vi "Timing Test.vi"() -> ()   [LabVIEW 2021]
uses:
  Ethernet/Ethernet.lvclass
  C:/Projects/1200-00006 _ BS1200/Engineering/Software/LabVIEW Driver/LV2021 Driver V2.0.0/BS1200 Driver/Battery Simulator 1200 Driver.lvclass
  CAN/CAN.lvclass
  Battery Simulator 1200 Driver.lvclass
panel:
  in  "Mode":enum16{"TCPIP", "CAN"}(ring)=enum."CAN"
  in  "CAN Interface":refnum<k21>="CAN1"
  out "Last update":timestamp
  in  "Stop Button":bool
  in  "UDP port":u16=54321
  in  "TCP port":u16=12345
  in  "Box IP address":string="192.168.1.100"
  in  "Update channel 1 voltage":dbl
  out "Array - String":string[](array[string])
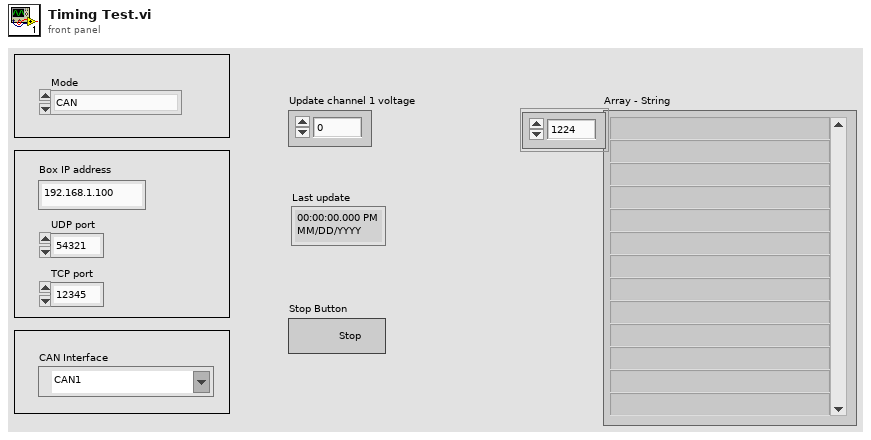
[diagram p1: front panel]
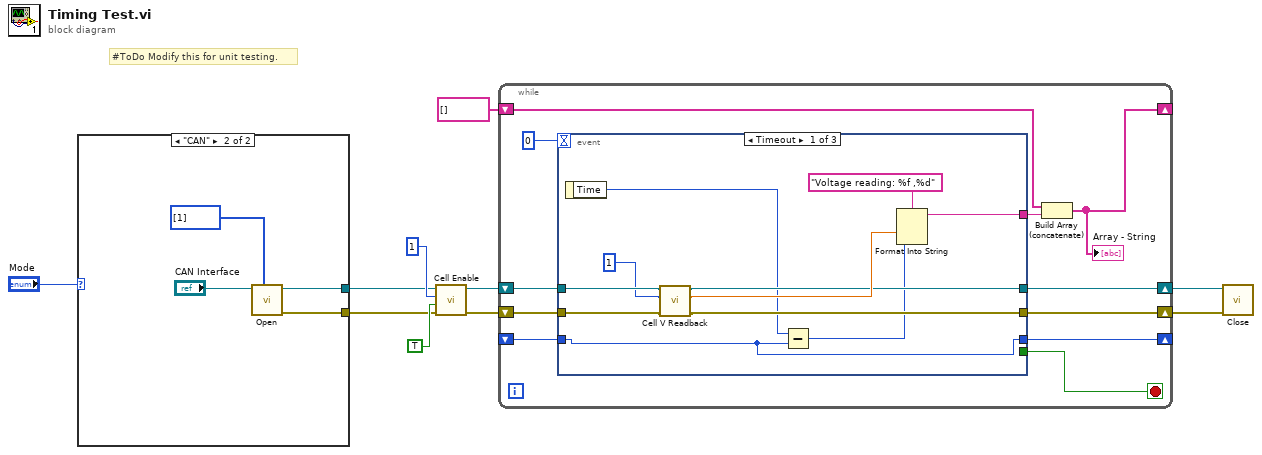
[diagram p0: block diagram]
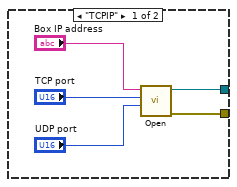
[diagram p2: hidden frame]
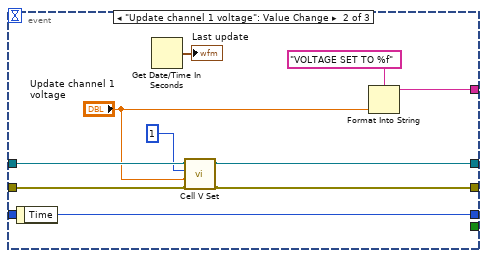
[diagram p3: hidden frame]
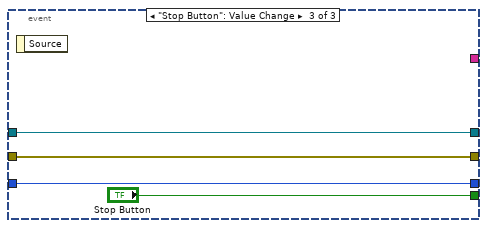
[diagram p4: hidden frame]
diagram:
  # "#ToDo Modify this for unit testing."
  n1 = case shown="\"CAN\"" "Mode" {
    tunnel: [w12 w19] -> w5
    tunnel: [w11 w18] -> w4
    frame "TCPIP" {
      n2 = call "Open.vi"("UDP port"="UDP port", "TCP port"="TCP port", "Box IP address"="Box IP address") -> ("error out"=w11:errorcluster, "ENET out"=w12:refnum<class "Ethernet.lvclass">)  [unwired: 7 in]
    }
    frame "CAN" {
      n3 = call "Open.vi"("Box IDs"=u8[] [1] ("Box ID Array"), "CAN Interface"="CAN Interface") -> ("error out"=w18:errorcluster, "CAN out"=w19:refnum<class "CAN.lvclass">)  [unwired: 8 in]
    }
  }
  n4 = call-dynamic "Cell Enable.vi"("error in (no error)"=w4, "Enable"=TRUE, "Channel"=u16 1, "Battery Simulator 1200 Driver in"=w5) -> ("error out"=w6:errorcluster, "Battery Simulator 1200 Driver out"=w7:refnum<class "Battery Simulator 1200 Driver.lvclass">)  [unwired: 6 in]
  n5 = while {
    shift-right: [w27] -> w3
    shift-left: w7 -> [w29]
    shift-right: [w28] -> w2
    shift-left: w6 -> [w26]
    shift-right: [w22] -> _
    shift-left: string[] [] -> [w23]
    shift-right: [w21] -> _
    shift-left: _ -> [w20]
    stop <- w25 stop-if-true
    n6 = event shown="[0] Timeout" {
      selector: _ -> [_ _ _]
      dyn-events: _ -> [_ _ _]
      timeout: 0 -> [_ _ _]
      tunnel: w29 -> [w35 w47 w54]
      tunnel: [w38 w48 w53] -> w28
      tunnel: [w36 w49 w54] -> w27
      tunnel: w26 -> [w39 w46 w53]
      tunnel: [_ _ "Stop Button"] -> w25
      tunnel: [w40 w50 _] -> w24
      tunnel: [w31 w42 w52] -> w21
      tunnel: w20 -> [w31 _ w52]
      event Timeout {
        n7 = event-data() -> ("Time"=w33:u32)  [unwired: 1 in]
        n8 = call-dynamic "Cell V Readback.vi"("error in (no error)"=w39, "Channel"=u16 1, "Battery Simulator 1200 Driver in"=w35) -> ("error out"=w38:errorcluster, "Voltage"=w37:dbl, "Battery Simulator 1200 Driver out"=w36:refnum<class "Battery Simulator 1200 Driver.lvclass">)  [unwired: 6 in]
        n9 = Subtract(x=w33, y=w31) -> (x-y=w32:u32)
        n10 = Format Into String(format string="Voltage reading: %f ,%d", w37, w32) -> (resulting string=w40:string)  [unwired: 2 in, 1 out]
      }
      event "Update channel 1 voltage": Value Change {
        n11 = event-data() -> ("Time"=w42:u32)  [unwired: 1 in]
        n12 = Get Date/Time In Seconds() -> (seconds since 1Jan1904=→"Last update":timestamp)
        n13 = call-dynamic "Cell V Set.vi"("error in (no error)"=w46, "Voltage"="Update channel 1 voltage", "Channel"=u16 1, "Battery Simulator 1200 Driver in"=w47) -> ("error out"=w48:errorcluster, "Battery Simulator 1200 Driver out"=w49:refnum<class "Battery Simulator 1200 Driver.lvclass">)  [unwired: 6 in]
        n14 = Format Into String(format string="VOLTAGE SET TO %f", "Update channel 1 voltage") -> (resulting string=w50:string)  [unwired: 2 in, 1 out]
      }
      event "Stop Button": Value Change {
        n15 = event-data() -> ()  [unwired: 1 in, 1 out]
      }
    }
    n16 = Build Array (concatenate)(w23, w24) -> (w22:string[])
    "Array - String" <- w22
  }
  n17 = call-dynamic "Close.vi"("error in (no error)"=w2, "Battery Simulator 1200 Driver in"=w3) -> ()  [unwired: 9 in, 1 out]
